vi "cv_03-01_random_check.vi"() -> ()   [LabVIEW 2013]
panel:
  in  "stop":bool
  out "# of iterations":u32
  out "Current Number":u16
  in  "Number to Match":u16 step=1
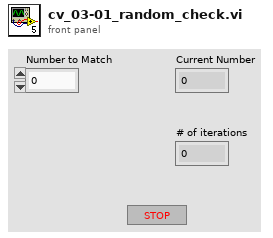
[diagram p1: front panel]
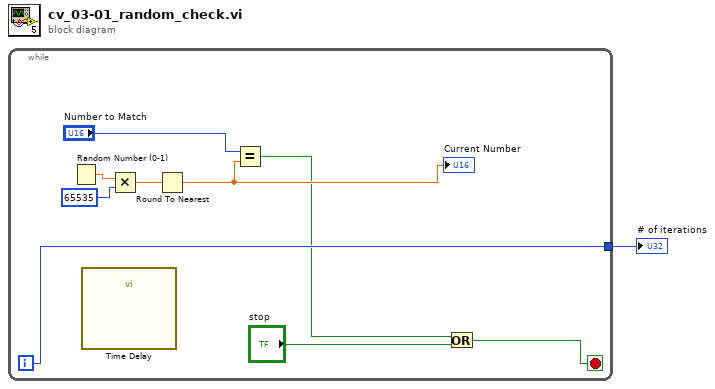
[diagram p0: block diagram]
diagram:
  n1 = while {
    tunnel: [w6] -> w1
    i -> [w6]
    stop <- w4 stop-if-true
    n2 = Random Number (0-1)() -> (number: 0 to 1=w10:dbl)
    n3 = call "Time Delay"() -> ()  [unwired: 11 in, 1 out]
    n4 = Multiply(x=w10, y=65535) -> (x*y=w8:dbl)
    n5 = Round To Nearest(number=w8) -> (nearest integer value=w5:dbl)
    "Current Number" <- w5
    n6 = Equal?(x="Number to Match", y=w5) -> (x = y?=w3:bool)
    n7 = Or(x=w3, y="stop") -> (x .or. y?=w4:bool)
  }
  "# of iterations" <- w1
